vi "Longueur d'onde.vi"(11 "T thermistances":dbl[](array[numeric])) -> (3 "Wavelenght":dbl format="%#_13g")   [LabVIEW 2018]
uses:
  <vilib>/Analysis/baseanly.llb/Mean (DBL).vi
  <vilib>/Analysis/NI_AALBase.lvlib
  <vilib>/gmath/NI_Gmath.lvlib
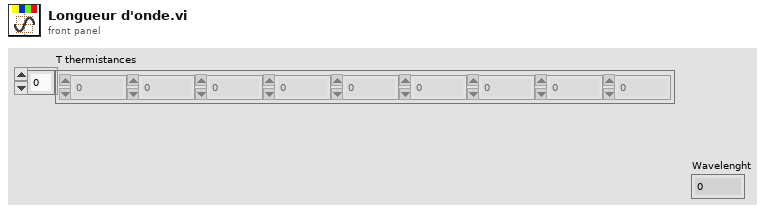
[diagram p1: front panel]
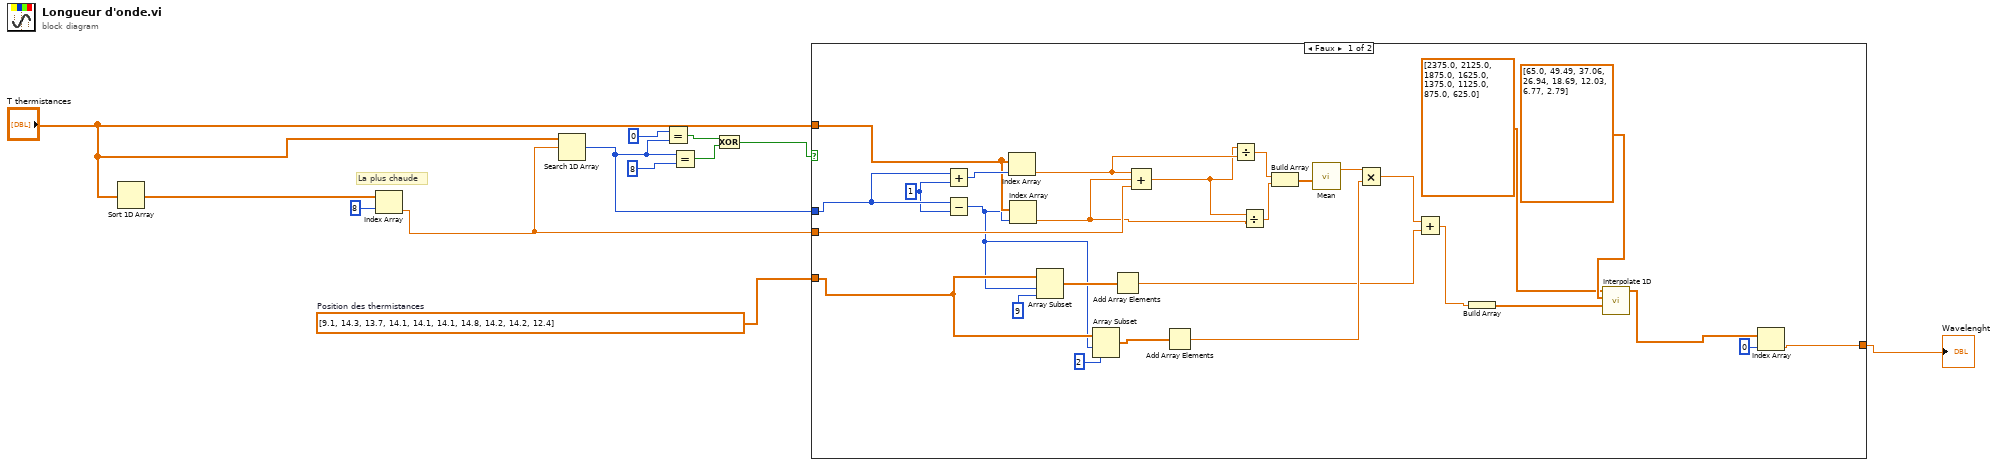
[diagram p0: block diagram]
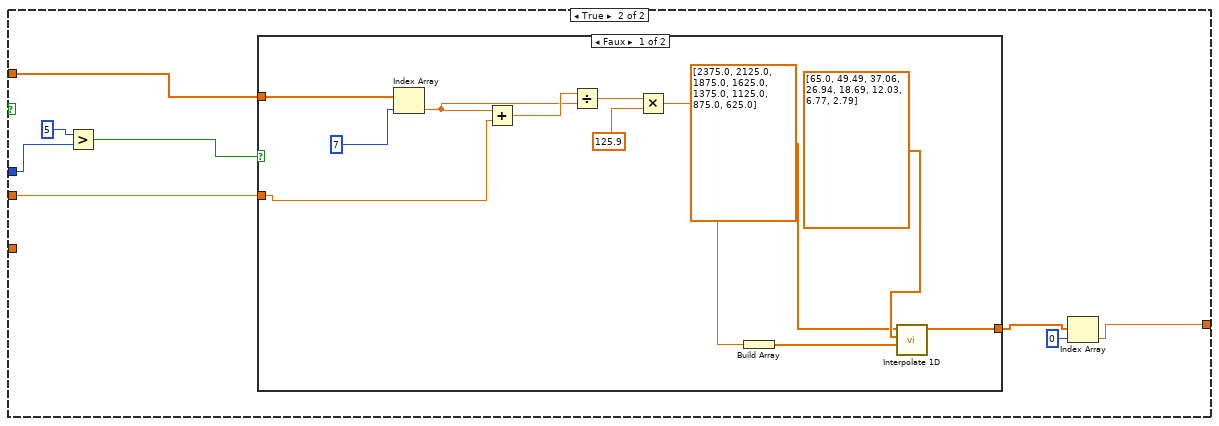
[diagram p2: hidden frame]
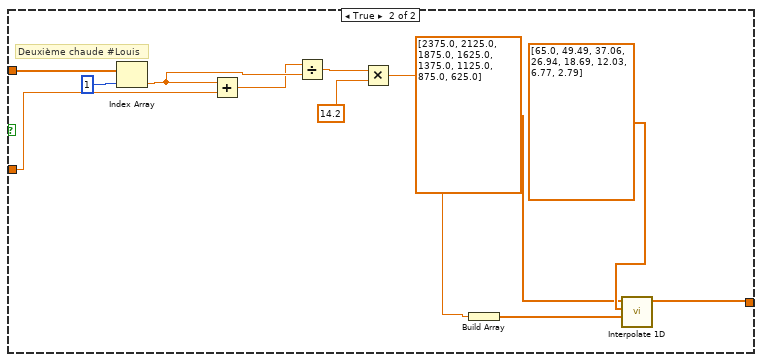
[diagram p3: hidden frame]
diagram:
  w2 = dbl[] [9.1, 14.3, 13.7, 14.1, 14.1, 14.1, 14.8, 14.2, 14.2, 12.4]  # Position des thermistances
  # "La plus chaude"
  n1 = Sort 1D Array(array="T thermistances") -> (sorted array=w11:dbl[])
  n2 = Index Array(array=w11, index=8 ("indice")) -> (element=w3:dbl)
  n3 = Search 1D Array(1D array="T thermistances", element=w3) -> (index of element=w8:i32)  [unwired: 1 in]
  n4 = Equal?(x=0, y=w8) -> (x = y?=w7:bool)
  n5 = Equal?(x=w8, y=8) -> (x = y?=w6:bool)
  n6 = Exclusive Or(1:w6, 2:w7) -> (0:w5:bool)
  n7 = case shown="Faux" w5 {
    tunnel: w8 -> [w40 w48]
    tunnel: "T thermistances" -> [w38 w45]
    tunnel: w3 -> [w36 w44]
    tunnel: w2 -> [w29 _]
    tunnel: [w13 w41] -> w1
    frame False {
      w37 = 1
      n8 = Add(x=w40, y=w37) -> (x+y=w39:i32)
      n9 = Subtract(x=w40, y=w37) -> (x-y=w27:i32)
      n10 = Index Array(array=w38, index=w39) -> (element=w18:dbl)
      n11 = Index Array(array=w38, index=w27) -> (element=w16:dbl)
      n12 = Array Subset(array=w29, index=w27, length=9) -> (w30:dbl[])
      n13 = Array Subset(array=w29, index=w27, length=2 ("longueur")) -> (w26:dbl[])
      n14 = Add Array Elements(numeric array=w30) -> (sum=w24:dbl)
      n15 = Compound Arithmetic op=ADD(w18, w16, w36) -> (w17:dbl)
      n16 = Add Array Elements(numeric array=w26) -> (sum=w25:dbl)
      n17 = Divide(x=w17, y=w18) -> (x/y=w34:dbl)
      n18 = Divide(x=w17, y=w16) -> (x/y=w35:dbl)
      n19 = Build Array(w34, w35) -> (w33:dbl[])
      n20 = call-poly <vilib>:"Mean.vi"("X"=w33) -> ("mean"=w31:dbl)  [unwired: 1 out]
      n21 = Multiply(x=w31, y=w25) -> (x*y=w23:dbl)
      n22 = Add(x=w23, y=w24) -> (x+y=w20:dbl)
      n23 = Build Array(w20) -> (w19:dbl[])
      n24 = call <vilib>:"Interpolate 1D.vi"("xi"=w19, "X"=dbl[] [65.0, 49.49, 37.06, 26.94, 18.69, 12.03, 6.77, 2.79], "Y"=dbl[] [2375.0, 2125.0, 1875.0, 1625.0, 1375.0, 1125.0, 875.0, 625.0]) -> ("yi"=w15:dbl[])  [unwired: 6 in, 2 out]
      n25 = Index Array(array=w15, index=0 ("indice")) -> (element=w13:dbl)
    }
    frame True {
      n26 = Greater?(x=5, y=w48) -> (0:w46:bool)
      n27 = case shown="Faux" w46 {
        tunnel: w45 -> [w59 w72]
        tunnel: w44 -> [w50 w71]
        tunnel: [w49 w61] -> w42
        frame False {
          n28 = Index Array(array=w59, index=7) -> (element=w51:dbl)
          n29 = Add(x=w51, y=w50) -> (x+y=w58:dbl)
          n30 = Divide(x=w58, y=w51) -> (x/y=w56:dbl)
          n31 = Multiply(x=w56, y=125.9) -> (x*y=w52:dbl)
          n32 = Build Array(w52) -> (w53:dbl[])
          n33 = call <vilib>:"Interpolate 1D.vi"("xi"=w53, "X"=dbl[] [65.0, 49.49, 37.06, 26.94, 18.69, 12.03, 6.77, 2.79], "Y"=dbl[] [2375.0, 2125.0, 1875.0, 1625.0, 1375.0, 1125.0, 875.0, 625.0]) -> ("yi"=w49:dbl[])  [unwired: 6 in, 2 out]
        }
        frame True {
          # "Deuxième chaude #Louis"
          n34 = Index Array(array=w72, index=1) -> (element=w69:dbl)
          n35 = Add(x=w69, y=w71) -> (x+y=w68:dbl)
          n36 = Divide(x=w68, y=w69) -> (x/y=w66:dbl)
          n37 = Multiply(x=w66, y=14.2) -> (x*y=w62:dbl)
          n38 = Build Array(w62) -> (w63:dbl[])
          n39 = call <vilib>:"Interpolate 1D.vi"("xi"=w63, "X"=dbl[] [65.0, 49.49, 37.06, 26.94, 18.69, 12.03, 6.77, 2.79], "Y"=dbl[] [2375.0, 2125.0, 1875.0, 1625.0, 1375.0, 1125.0, 875.0, 625.0]) -> ("yi"=w61:dbl[])  [unwired: 6 in, 2 out]
        }
      }
      n40 = Index Array(array=w42, index=0 ("indice")) -> (element=w41:dbl)
    }
  }
  "Wavelenght" <- w1
